vi "Create Event References.vi"(8 "error in (no error)":errorcluster, 11 "Engine in":refnum<class "Engine.lvclass">) -> (0 "error out":errorcluster, 3 "Engine out":refnum<class "Engine.lvclass">)   [LabVIEW 2019, in "Engine.lvlib" / "Engine.lvclass"]
doc: "This routine creates events references. It should only be called when the initialization being performed is the root actor. (<b>IsRoot == TRUE</b>)"
uses:
  Project/Engine.lvclass
  Custom Controls/System Status.ctl
  Project/Engine.lvclass/Engine.ctl
  builds/Tools/QDMH.lvlibp/QDMH.lvclass
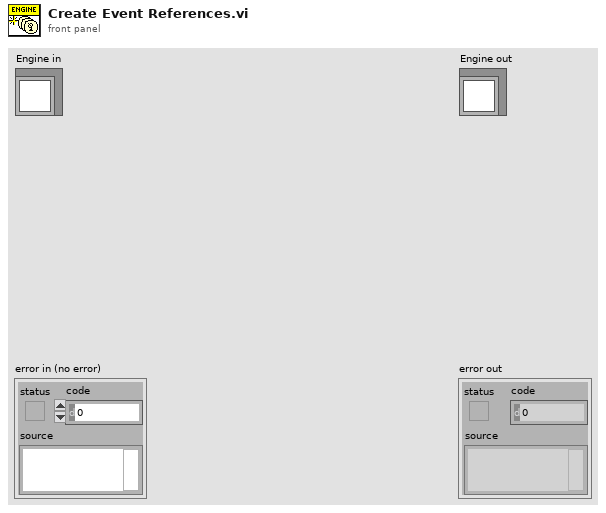
[diagram p1: front panel]
types:
  T1 = typedef "Engine.lvlib/Engine.lvclass/System Status.ctl" = enum16{"Logged Off", "UUT_Info_Missing", "Idle", "Error", "Warning", "Loading", "Config", "Manual", "Automation", "Report_View", "Previous"}
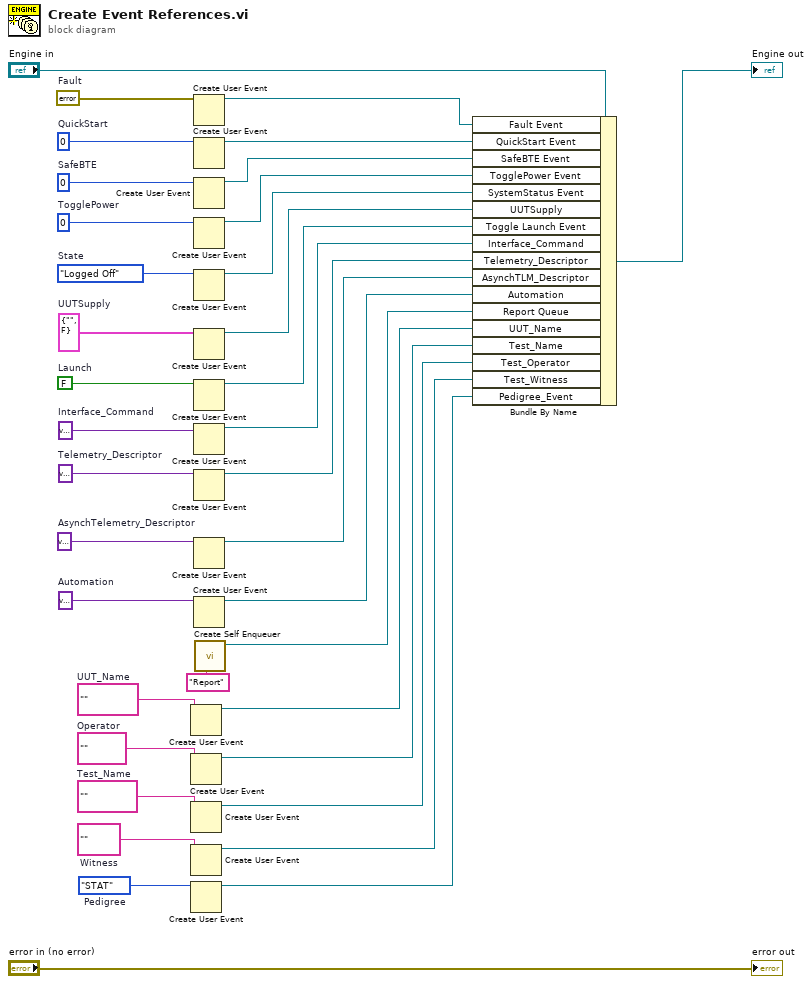
[diagram p0: block diagram]
diagram:
  w10 = enum16{"STAT", "BB", "PT", "EM", "FT"}."STAT"  # Pedigree
  w9 = ""  # Witness
  w8 = ""  # Test_Name
  w7 = ""  # Operator
  w6 = ""  # UUT_Name
  w13 = System_Status."Logged Off"  # State
  w29 = variant  # Automation
  w28 = variant  # AsynchTelemetry_Descriptor
  w27 = variant  # Telemetry_Descriptor
  w26 = variant  # Interface_Command
  w25 = FALSE  # Launch
  w30 = cluster{"Supply":string, "Output":bool} {"Supply"="", "Output"=FALSE}  # UUTSupply
  w34 = 0  # TogglePower
  w33 = 0  # SafeBTE
  w32 = 0  # QuickStart
  w31 = errorcluster {"status"=FALSE, "code"=0, "source"=""}  # Fault
  n1 = Create User Event(user event datatype=w6) -> (user event=w5:refnum<user-event>)  [unwired: 1 in, 1 out]
  n2 = Create User Event(user event datatype=w7) -> (user event=w4:refnum<user-event>)  [unwired: 1 in, 1 out]
  n3 = Create User Event(user event datatype=w8) -> (user event=w3:refnum<user-event>)  [unwired: 1 in, 1 out]
  n4 = Create User Event(user event datatype=w9) -> (user event=w2:refnum<user-event>)  [unwired: 1 in, 1 out]
  n5 = Create User Event(user event datatype=w10) -> (user event=w1:refnum<user-event>)  [unwired: 1 in, 1 out]
  n6 = Create User Event(user event datatype=w31) -> (user event=w24:refnum<user-event>)  [unwired: 1 in, 1 out]
  n7 = Create User Event(user event datatype=w32) -> (user event=w23:refnum<user-event>)  [unwired: 1 in, 1 out]
  n8 = Create User Event(user event datatype=w33) -> (user event=w22:refnum<user-event>)  [unwired: 1 in, 1 out]
  n9 = Create User Event(user event datatype=w34) -> (user event=w21:refnum<user-event>)  [unwired: 1 in, 1 out]
  n10 = Create User Event(user event datatype=w13) -> (user event=w20:refnum<user-event>)  [unwired: 1 in, 1 out]
  n11 = Create User Event(user event datatype=w30) -> (user event=w19:refnum<user-event>)  [unwired: 1 in, 1 out]
  n12 = Create User Event(user event datatype=w25) -> (user event=w18:refnum<user-event>)  [unwired: 1 in, 1 out]
  n13 = Create User Event(user event datatype=w26) -> (user event=w17:refnum<user-event>)  [unwired: 1 in, 1 out]
  n14 = Create User Event(user event datatype=w27) -> (user event=w16:refnum<user-event>)  [unwired: 1 in, 1 out]
  n15 = Create User Event(user event datatype=w28) -> (user event=w15:refnum<user-event>)  [unwired: 1 in, 1 out]
  n16 = Create User Event(user event datatype=w29) -> (user event=w14:refnum<user-event>)  [unwired: 1 in, 1 out]
  n17 = call "Create Self Enqueuer.vi"("Name"="Report") -> ("QDMH out"=w11:refnum<class "QDMH.lvclass">)  [unwired: 9 in, 1 out]
  n18 = Bundle By Name(cluster="Engine in", "Fault Event"=w24, "QuickStart Event"=w23, "SafeBTE Event"=w22, "TogglePower Event"=w21, "SystemStatus Event"=w20, "UUTSupply"=w19, "Toggle Launch Event"=w18, "Interface_Command"=w17, "Telemetry_Descriptor"=w16, "AsynchTLM_Descriptor"=w15, "Automation"=w14, "Report Queue"=w11, "UUT_Name"=w5, "Test_Name"=w4, "Test_Operator"=w3, "Test_Witness"=w2, "Pedigree_Event"=w1) -> (→"Engine out":refnum<class "Engine.lvclass">)
  "error out" <- "error in (no error)"
